vi "Digitizer Limit Check.vi"(7 "VI Action":T1=enum."Write", 8 "Index":i32, 9 "Lower Limit":dbl, 10 "Upper Limit":dbl, 11 "X":dbl[](array[numeric]) format="%0.2f") -> (3 "Array":bool[](array[boolean]))   [LabVIEW 2010]
uses:
  status action.ctl
  <vilib>/Analysis/5stat.llb/RMS (DBL).vi
  <vilib>/Analysis/NI_AALPro.lvlib
panel:
  out "In Range?":bool
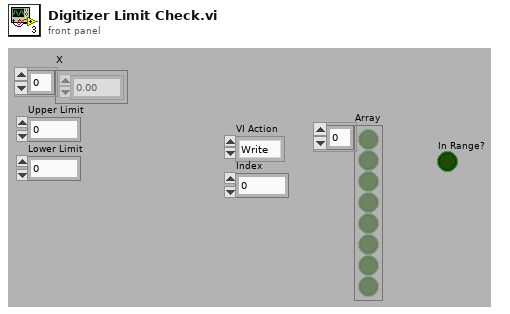
[diagram p1: front panel]
types:
  T1 = typedef "status action.ctl" = enum16{"Initialize", "Write", "Read"}
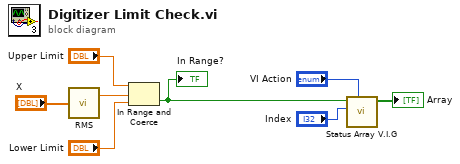
[diagram p0: block diagram]
diagram:
  n1 = call-poly <vilib>:"RMS.vi"("X"="X") -> ("rms value"=w5:dbl)  [unwired: 1 out]
  n2 = In Range and Coerce(upper limit="Upper Limit", x=w5, lower limit="Lower Limit") -> (In Range?=w1:bool)  [unwired: 1 out]
  "In Range?" <- w1
  n3 = call "Status Array V.I.G.vi"("VI Action"="VI Action", "index"="Index", "Element"=w1) -> ("Array"=→"Array":bool[])  [unwired: 8 in]
